vi "sequences.vi"(0 "sequence":T6=enum."warmup", 7 "sequenzen":T2, 11 "command parameter":T3={"CO2 ref"=392.0, "CO2 span"=372.0, "H2O ref"=0.0, "H2O span"=0.0, "Zi"=0.0, "Zt"=1.2, "Zm"=0.0, "S"=0.0, "Temp [C]"=50.0, "Pressure [hPa]"=135.0, "Licor-Sources"=["CO2A W", "CO2B W", "H2OA W", "H2OB W", "T C", "T V", "P kPa", "P V", "RH %", "CO2A um/m", "CO2B um/m", "H2OA mm/m", "H2OB mm/m"], "Licor-Pump"="Off", "Zeitstempel"=timestamp(0 s since 1904-01-01)} {"Pressure [hPa]" format="%_5g"; "Temp [C]" format="%.2f"; "CO2 ref" format="%.2f"; "CO2 span" format="%.2g"; "H2O ref" format="%.2g"; "H2O span" format="%.2g"; "Zt" format="%#_4g"}) -> (8 "sequence out":cluster{"time":i32, "command":string}[](array[cluster]))   [LabVIEW 2010, in "Licor-Steuerung.lvlib"]
uses:
  Licor-Steuerung.lvlib
  Licor-Sequences.ctl
  Licor-Parameter.ctl
  LicorLI7000/conventions/Licor-Source.ctl
  Licor-Pump.ctl
  Licor-Commands.ctl
  LicorLI7000/LicorLI7000.lvlib
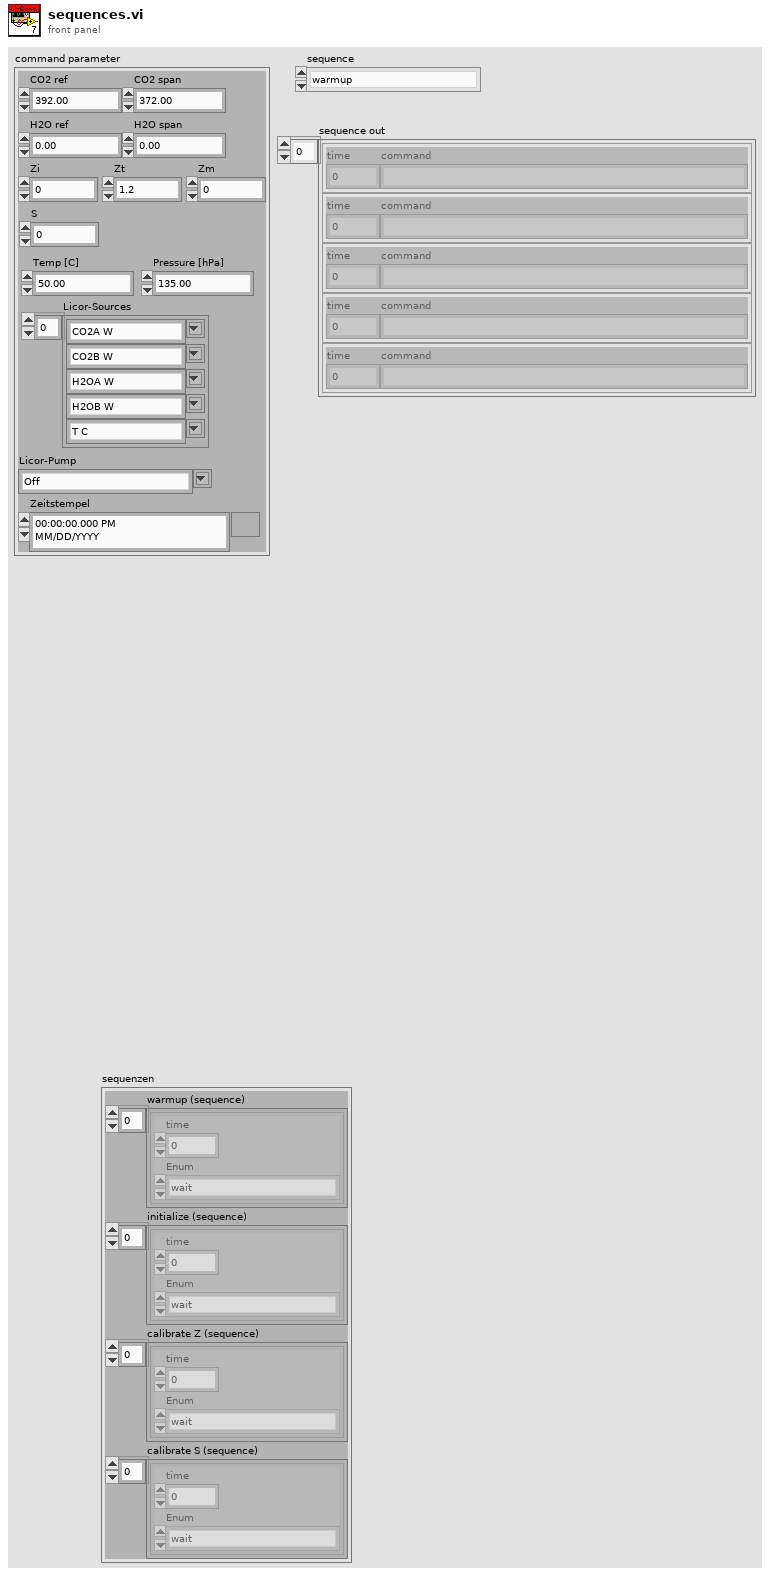
[diagram p1: front panel]
types:
  T1 = typedef "Licor-Steuerung.lvlib/Licor-Commands.ctl" = enum16{"wait", "initialize", "resetCO2", "resetH2O", "getReference", "setReference", "calibration-Z-CO2", "calibration-Z-H2O", "calibration-S-CO2", "calibration-S-H2O", "getCalibrationParameter", "setZeroParameter", "setLicorTime", "getLicorTime", "setPumpFlowrate", "setPumpSlow", "setPumpMedium", "setPumpFast", "getInfo"}
  T2 = cluster{"warmup (sequence)":cluster{"time":i32, "Enum":T1}[], "initialize (sequence)":cluster{"time":i32, "Enum":T1}[], "calibrate Z (sequence)":cluster{"time":i32, "Enum":T1}[], "calibrate S (sequence)":cluster{"time":i32, "Enum":T1}[]}
  T3 = typedef "Licor-Steuerung.lvlib/Licor-Parameter.ctl" = cluster{"CO2 ref":dbl, "CO2 span":dbl, "H2O ref":dbl, "H2O span":dbl, "Zi":dbl, "Zt":dbl, "Zm":dbl, "S":dbl, "Temp [C]":dbl, "Pressure [hPa]":dbl, "Licor-Sources":T4[], "Licor-Pump":T5, "Zeitstempel":timestamp}
  T4 = typedef "LicorLI7000.lvlib/Licor-Source.ctl" = string
  T5 = typedef "Licor-Steuerung.lvlib/Licor-Pump.ctl" = string
  T6 = typedef "Licor-Steuerung.lvlib/Licor-Sequences.ctl" = enum16{"test", "WAIT", "warmup", "initialize", "calibrate Z", "calibrate S"}
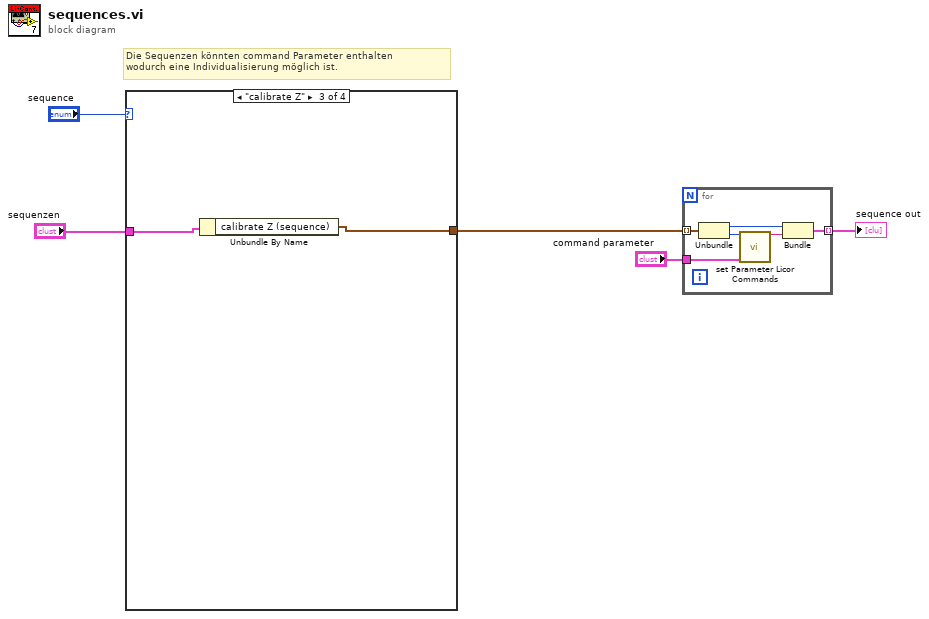
[diagram p0: block diagram]
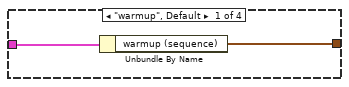
[diagram p2: hidden frame]
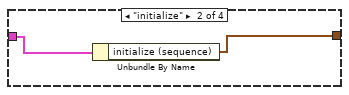
[diagram p3: hidden frame]
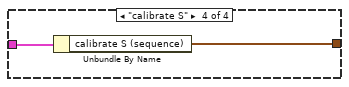
[diagram p4: hidden frame]
diagram:
  # "Die Sequenzen könnten command Parameter enthalten \nwodurch eine Individualisierung möglich ist."
  n1 = case shown="\"calibrate Z\"" "sequence" {
    tunnel: [w6 w8 w10 w12] -> w5
    tunnel: "sequenzen" -> [w7 w9 w11 w13]
    frame "warmup", Default {
      n2 = Unbundle By Name(w7) -> ("warmup (sequence)"=w6:cluster{"time":i32, "Enum":T1}[])
    }
    frame "initialize" {
      n3 = Unbundle By Name(w9) -> ("initialize (sequence)"=w8:cluster{"time":i32, "Enum":T1}[])
    }
    frame "calibrate Z" {
      n4 = Unbundle By Name(w11) -> ("calibrate Z (sequence)"=w10:cluster{"time":i32, "Enum":T1}[])
    }
    frame "calibrate S" {
      n5 = Unbundle By Name(w13) -> ("calibrate S (sequence)"=w12:cluster{"time":i32, "Enum":T1}[])
    }
  }
  n6 = for {
    tunnel: w5 -> [w19] mode=indexing
    tunnel: "command parameter" -> [w17]
    tunnel: [w14] -> w4 mode=indexing
    n7 = Unbundle(w19) -> ("time"=w16:i32, "Enum"=w18:T1)
    n8 = call "set Parameter Licor Commands.vi"("Licor-Commands"=w18, "command parameter"=w17) -> ("command"=w15:string)  [unwired: 13 in]
    n9 = Bundle("time"=w16, "command"=w15) -> (w14:cluster{"time":i32, "command":string})  [unwired: 1 in]
  }
  "sequence out" <- w4
